vi "Get SMO HELP getAll.vi"(8 "error in (no error)":errorcluster, 11 "Inst.FP in":refnum<class "Inst.FP.lvclass">) -> (0 "error out":errorcluster, 2 "response cluster":variant, 3 "Inst.FP out":refnum<class "Inst.FP.lvclass">)   [LabVIEW 2019, in "Inst.FP.lvclass"]
uses:
  Inst.FP.lvclass
  <userlib>/LevyLab/Instrument Framework/Instrument Types/Cryostat/Instrument.Cryostat.lvclass
  Typedefs/Inst.FP.getAll--Cluster.ctl
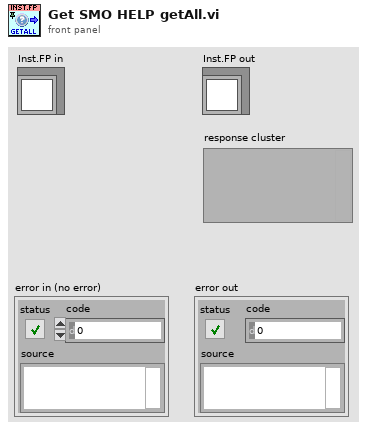
[diagram p1: front panel]
types:
  T1 = typedef "Inst.FP.lvclass/Inst.FP.getAll--Cluster.ctl" = cluster{"FP Data":dbl[], "MG Data":dbl[], "PT Data":dbl[], "Status Array":u32[], "Mode":string}
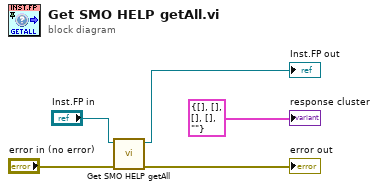
[diagram p0: block diagram]
diagram:
  n1 = call-parent "Get SMO HELP getAll.vi"("error in (no error)"="error in (no error)", "Instrument in"="Inst.FP in") -> ("error out"=→"error out":errorcluster, "Instrument out"=→"Inst.FP out":refnum<class "Inst.FP.lvclass">)  [unwired: 7 in, 1 out]
  "response cluster" <- T1 {"FP Data"=[], "MG Data"=[], "PT Data"=[], "Status Array"=[], "Mode"=""} ("getAll")
